vi "Files_not_found_warning.vi"(2 "Use Selected Folder?":bool, 3 "Total number of data files":i32, 4 "Unfound Files":path[](array[path])) -> (0 "Edit Selected Folder Out":bool, 1 "Edit Files?":bool)   [LabVIEW 2010]
panel:
  in  "Edit Selected Folder":bool
  in  "Cancel":bool
  in  "Edit files that have been found?":bool
  out "Message":string
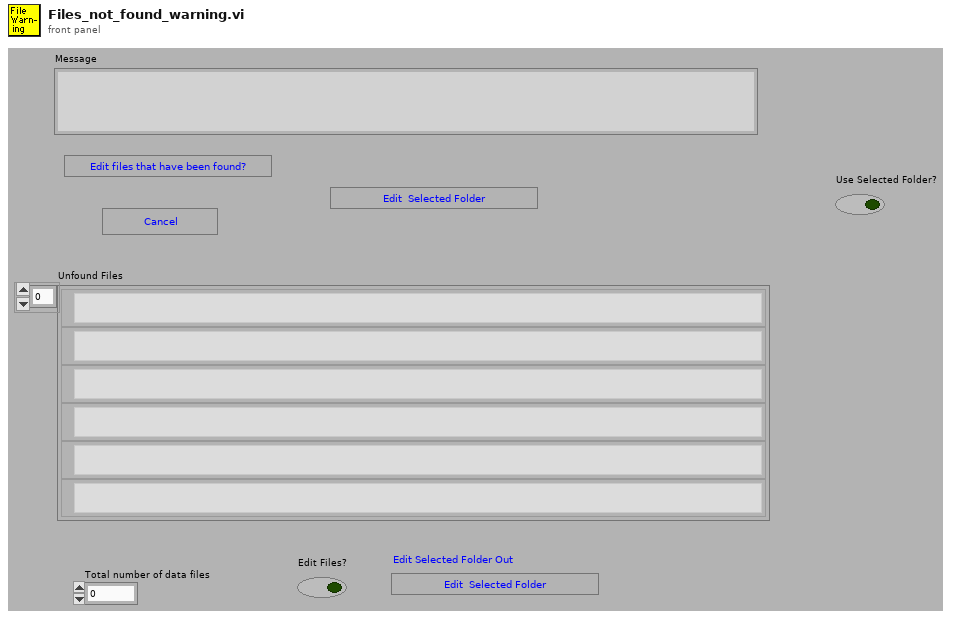
[diagram p1: front panel]
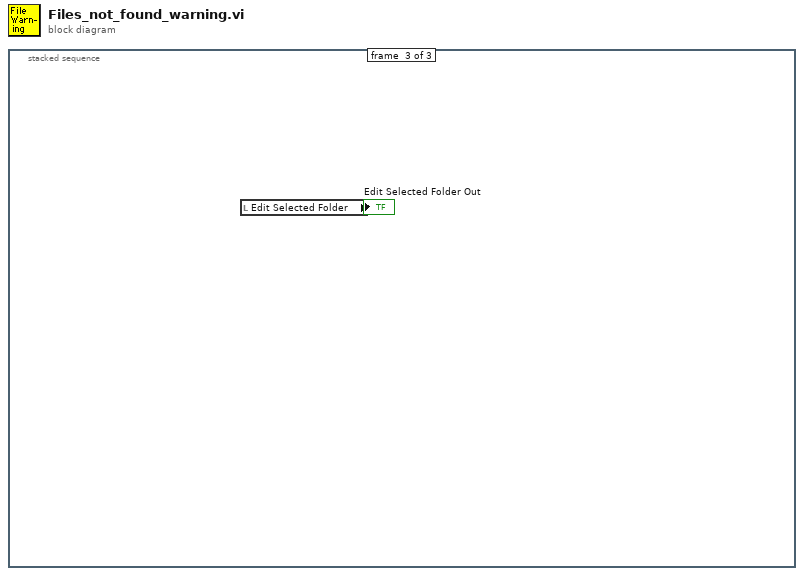
[diagram p0: block diagram]
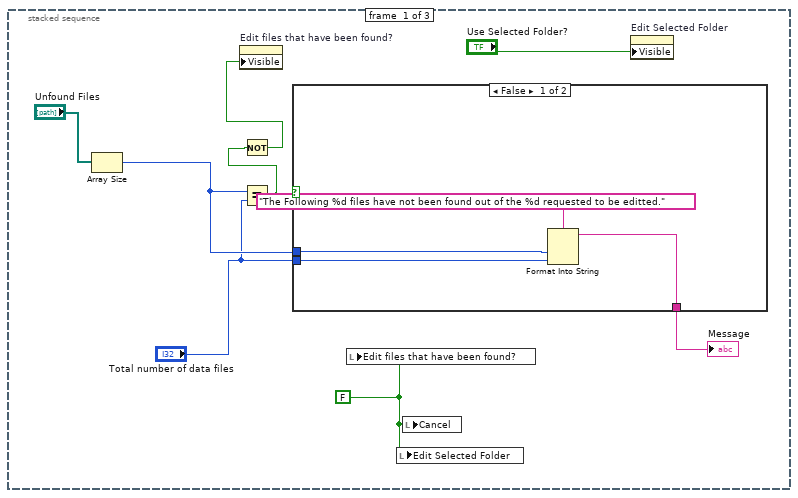
[diagram p2: hidden frame]
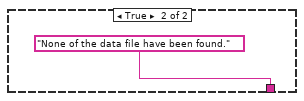
[diagram p3: hidden frame]
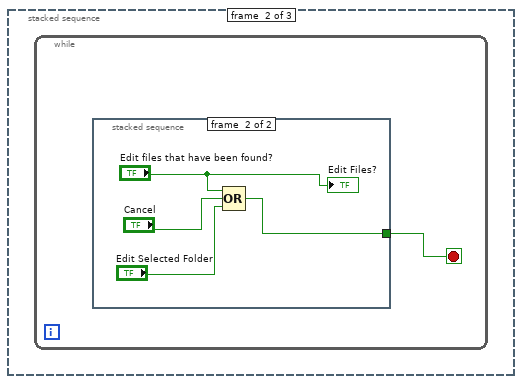
[diagram p4: hidden frame]
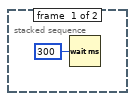
[diagram p5: hidden frame]
diagram:
  n1 = stacked-sequence {
    frame #0 {
      w2 = FALSE ("Edit files")
      n2 = Array Size(array="Unfound Files") -> (size(s)=w7:i32)
      n3 = Equal?(x=w7, y="Total number of data files") -> (x = y?=w4:bool)
      n4 = Not(x=w4) -> (.not. x?=w3:bool)
      n5 = property on="Edit files that have been found?" class="Bool (strict)"("Visible"=w3) -> ()  [unwired: 2 in, 2 out]
      n6 = case shown="False" w4 {
        tunnel: w7 -> [w11 _]
        tunnel: "Total number of data files" -> [w10 _]
        tunnel: [w9 "None of the data file have been found."] -> w5
        frame False {
          n7 = Format Into String(format string="The Following %d files have not been found out of the %d requested to be editted.", w11, w10) -> (resulting string=w9:string)  [unwired: 2 in, 1 out]
        }
        frame True {
        }
      }
      "Message" <- w5
      n8 = local write "Edit files that have been found?"(w2) -> ()
      n9 = local write "Edit Selected Folder"(w2) -> ()
      n10 = local write "Cancel"(w2) -> ()
      n11 = property on="Edit Selected Folder" class="Bool (strict)"("Visible"="Use Selected Folder?") -> ()  [unwired: 2 in, 2 out]
    }
    frame #1 {
      n12 = while {
        stop <- w14 stop-if-true
        n13 = stacked-sequence {
          tunnel: [_ w18] -> w14
          frame #0 {
            n14 = Wait (ms)(milliseconds to wait=u32 300) -> ()  [unwired: 1 out]
          }
          frame #1 {
            n15 = Compound Arithmetic op=OR("Edit files that have been found?", "Cancel", "Edit Selected Folder") -> (w18:bool)
            "Edit Files?" <- "Edit files that have been found?"
          }
        }
      }
    }
    frame #2 {
      n16 = local read "Edit Selected Folder"() -> (→"Edit Selected Folder Out":bool)
    }
  }
